vi "Change Query Conditions from Disp to TDM names.vi"(8 "error in (no error)":errorcluster, 10 "Conditions":T4[](array[typedef]), 11 "System Fields (none)":T1[](array[typedef])) -> (0 "error out":errorcluster, 2 "Array":T4[](array[typedef]))   [LabVIEW 2011]
uses:
  Datafinder Query.ctl
  eSearch Types.ctl
  DataFinder Comparisons.ctl
  database/Fields/Field Record.ctl
  database/Fields/Field DataTypes.ctl
  database/Fields/Field NextItem.ctl
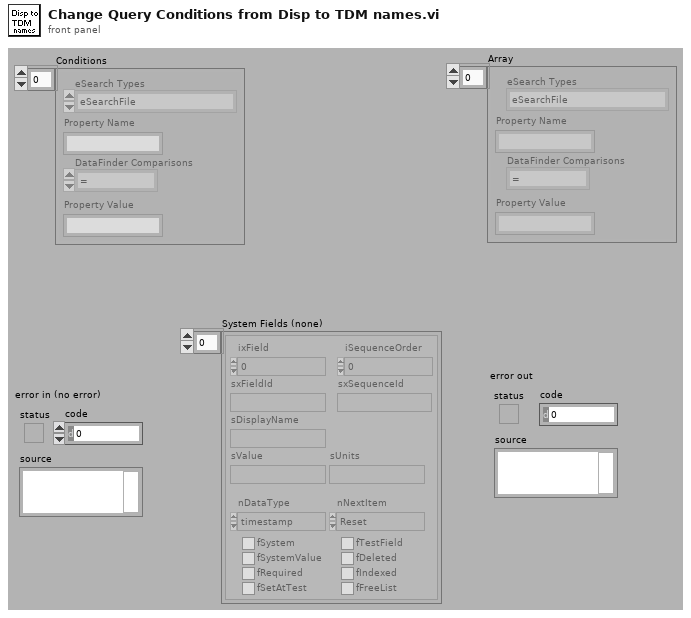
[diagram p1: front panel]
types:
  T1 = typedef "Field Record.ctl" = cluster{"ixField":i32, "iSequenceOrder":i32, "sxFieldId":string, "sxSequenceId":string, "sDisplayName":string, "sValue":string, "sUnits":string, "nDataType":T2, "nNextItem":T3, "fSystem":bool, "fSystemValue":bool, "fRequired":bool, "fSetAtTest":bool, "fTestField":bool, "fDeleted":bool, "fIndexed":bool, "fFreeList":bool}
  T2 = typedef "Field DataTypes.ctl" = enum32{"text", "numeric", "list", "timestamp", "boolean"}
  T3 = typedef "Field NextItem.ctl" = enum32{"Reset", "Retain", "Auto-Increment"}
  T4 = typedef "Datafinder Query.ctl" = cluster{"eSearch Types":T5, "Property Name":string, "DataFinder Comparisons":T6, "Property Value":string}
  T5 = typedef "eSearch Types.ctl" = enum16{"eSearchFile", "eSearchChannelGroup", "eSearchChannel"}
  T6 = typedef "DataFinder Comparisons.ctl" = enum16{"=", "<>", "<", "<=", ">", ">="}
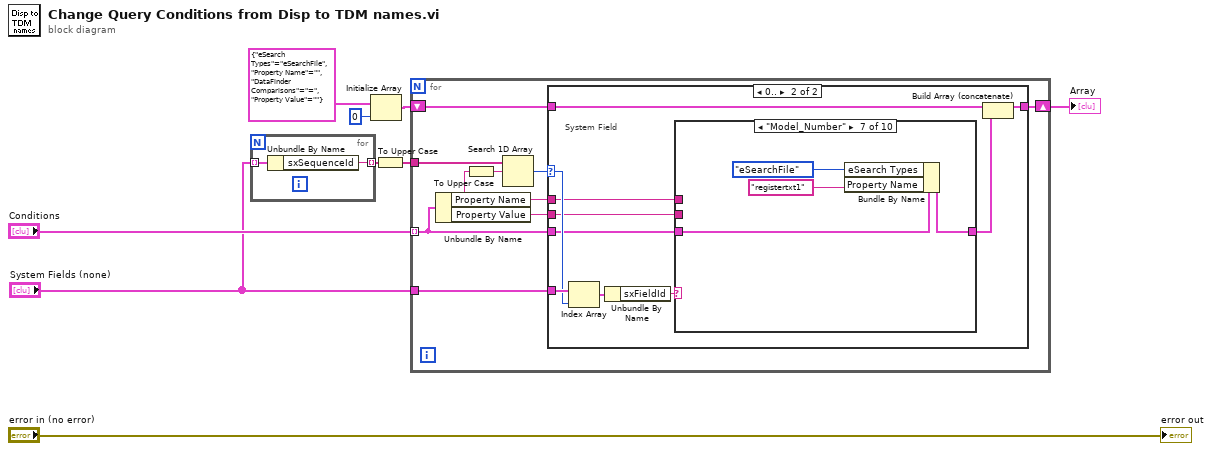
[diagram p0: block diagram]
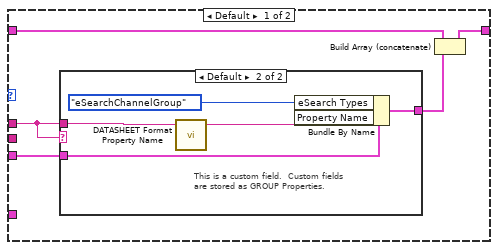
[diagram p2: hidden frame]
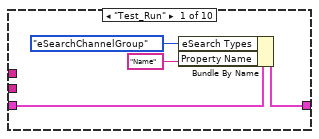
[diagram p4: hidden frame]
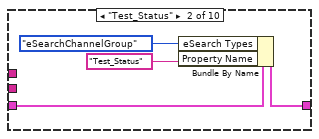
[diagram p5: hidden frame]
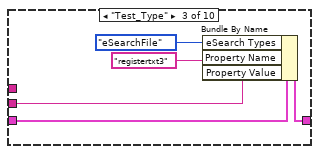
[diagram p6: hidden frame]
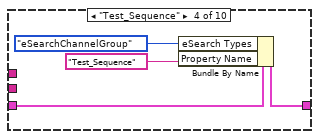
[diagram p7: hidden frame]
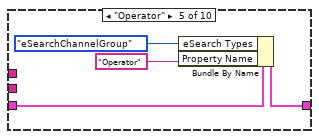
[diagram p8: hidden frame]
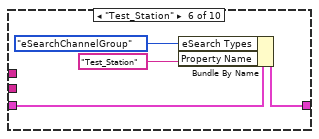
[diagram p9: hidden frame]
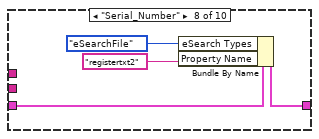
[diagram p10: hidden frame]
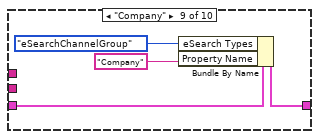
[diagram p11: hidden frame]
diagram:
  n1 = for {
    tunnel: "System Fields (none)" -> [w11] mode=indexing
    tunnel: [w10] -> w4 mode=indexing
    n2 = Unbundle By Name(w11) -> ("sxSequenceId"=w10:string)
  }
  n3 = Initialize Array(T4 {"eSearch Types"=enum."eSearchFile", "Property Name"="", "DataFinder Comparisons"=enum."=", "Property Value"=""} ("Data Finder Parameters"), 0 ("dimension size")) -> (w5:T4[])
  n4 = To Upper Case(1:w4) -> (0:w3:string[])
  n5 = for {
    tunnel: "Conditions" -> [w16] mode=indexing
    tunnel: w3 -> [w20]
    tunnel: "System Fields (none)" -> [w17]
    shift-right: [w15] -> w9
    shift-left: w5 -> [w18]
    n6 = Unbundle By Name(w16) -> ("Property Name"=w14:string, "Property Value"=w12:string)
    n7 = To Upper Case(1:w14) -> (0:w13:string)
    n8 = Search 1D Array(1D array=w20, element=w13) -> (index of element=w19:i32)  [unwired: 1 out]
    n9 = case shown="0.." w19 {
      selector: w19 -> [_ w40]
      tunnel: w18 -> [w25 w37]
      tunnel: [w24 w38] -> w15
      tunnel: w17 -> [_ w41]
      tunnel: w16 -> [w23 w35]
      tunnel: w14 -> [w21 w33]
      tunnel: w12 -> [_ w32]
      frame Default {
        n10 = case shown="Default" w21 {
          tunnel: w23 -> [w26 w31]
          tunnel: [w26 w30] -> w22
          tunnel: w21 -> [_ w28]
          frame "Model_Number", "Serial_Number", "Test_Type" {
            # "Trap case of special nongroup conditions"
          }
          frame Default {
            # "This is a custom field.  Custom fields\nare stored as GROUP Properties."
            n11 = call "DATASHEET Format Property Name.vi"("String with \\r or \\n"=w28) -> ("String without \\r or \\n"=w27:string)  [unwired: 4 out]
            n12 = Bundle By Name(cluster=w31, "eSearch Types"=eSearch_Types."eSearchChannelGroup", "Property Name"=w27) -> (w30:T4)
          }
        }
        n13 = Build Array (concatenate)(w25, w22) -> (w24:T4[])
      }
      frame 0.. {
        # "System Field"
        n14 = Index Array(array=w41, index=w40) -> (element=w39:T1)
        n15 = Unbundle By Name(w39) -> ("sxFieldId"=w36:string)
        n16 = case shown="\"Model_Number\"" w36 {
          tunnel: w35 -> [w45 w49 w51 w58 w62 w66 w70 w74 w78 w79]
          tunnel: [w44 w48 w54 w57 w61 w65 w69 w73 w77 w79] -> w34
          tunnel: w33 -> [_ _ _ _ _ _ _ _ _ _]
          tunnel: w32 -> [_ _ w50 _ _ _ _ _ _ _]
          frame "Test_Run" {
            n17 = Bundle By Name(cluster=w45, "eSearch Types"=eSearch_Types."eSearchChannelGroup", "Property Name"="Name") -> (w44:T4)
          }
          frame "Test_Status" {
            n18 = Bundle By Name(cluster=w49, "eSearch Types"=eSearch_Types."eSearchChannelGroup", "Property Name"="Test_Status") -> (w48:T4)
          }
          frame "Test_Type" {
            n19 = Bundle By Name(cluster=w51, "eSearch Types"=eSearch_Types."eSearchFile", "Property Name"="registertxt3", "Property Value"=w50) -> (w54:T4)
          }
          frame "Test_Sequence" {
            n20 = Bundle By Name(cluster=w58, "eSearch Types"=eSearch_Types."eSearchChannelGroup", "Property Name"="Test_Sequence") -> (w57:T4)
          }
          frame "Operator" {
            n21 = Bundle By Name(cluster=w62, "eSearch Types"=eSearch_Types."eSearchChannelGroup", "Property Name"="Operator") -> (w61:T4)
          }
          frame "Test_Station" {
            n22 = Bundle By Name(cluster=w66, "eSearch Types"=eSearch_Types."eSearchChannelGroup", "Property Name"="Test_Station") -> (w65:T4)
          }
          frame "Model_Number" {
            n23 = Bundle By Name(cluster=w70, "eSearch Types"=eSearch_Types."eSearchFile", "Property Name"="registertxt1") -> (w69:T4)
          }
          frame "Serial_Number" {
            n24 = Bundle By Name(cluster=w74, "eSearch Types"=eSearch_Types."eSearchFile", "Property Name"="registertxt2") -> (w73:T4)
          }
          frame "Company" {
            n25 = Bundle By Name(cluster=w78, "eSearch Types"=eSearch_Types."eSearchChannelGroup", "Property Name"="Company") -> (w77:T4)
          }
          frame Default {
            # "Don't know what this is  Just\npass it on through."
          }
        }
        n26 = Build Array (concatenate)(w37, w34) -> (w38:T4[])
      }
    }
  }
  "Array" <- w9
  "error out" <- "error in (no error)"
